vi "Close.vi"(8 "error in (no error)":errorcluster) -> (0 "error out":errorcluster)   [LabVIEW 2018, in "app_log.lvlib"]
doc: "Closes the reference to the log file.\n\nError handling\n- execute even if error at input\n- clear all errors (i.e. guaranteed that this VI will NOT generate an error of its own)\n- pass error in to error out"
uses:
  app_log.lvlib
  text_file/text_file.lvlib
panel:
  # "Development\ncontrols/indicators useful for development and testing, but which are not outputs of the VI"
  # "Input\nInputs to the VI"
  # "Output\nOutputs of the VI"
  # "Description\n\nBlank VI with error handling case. \n\nSummarize the use of this VI in this space."
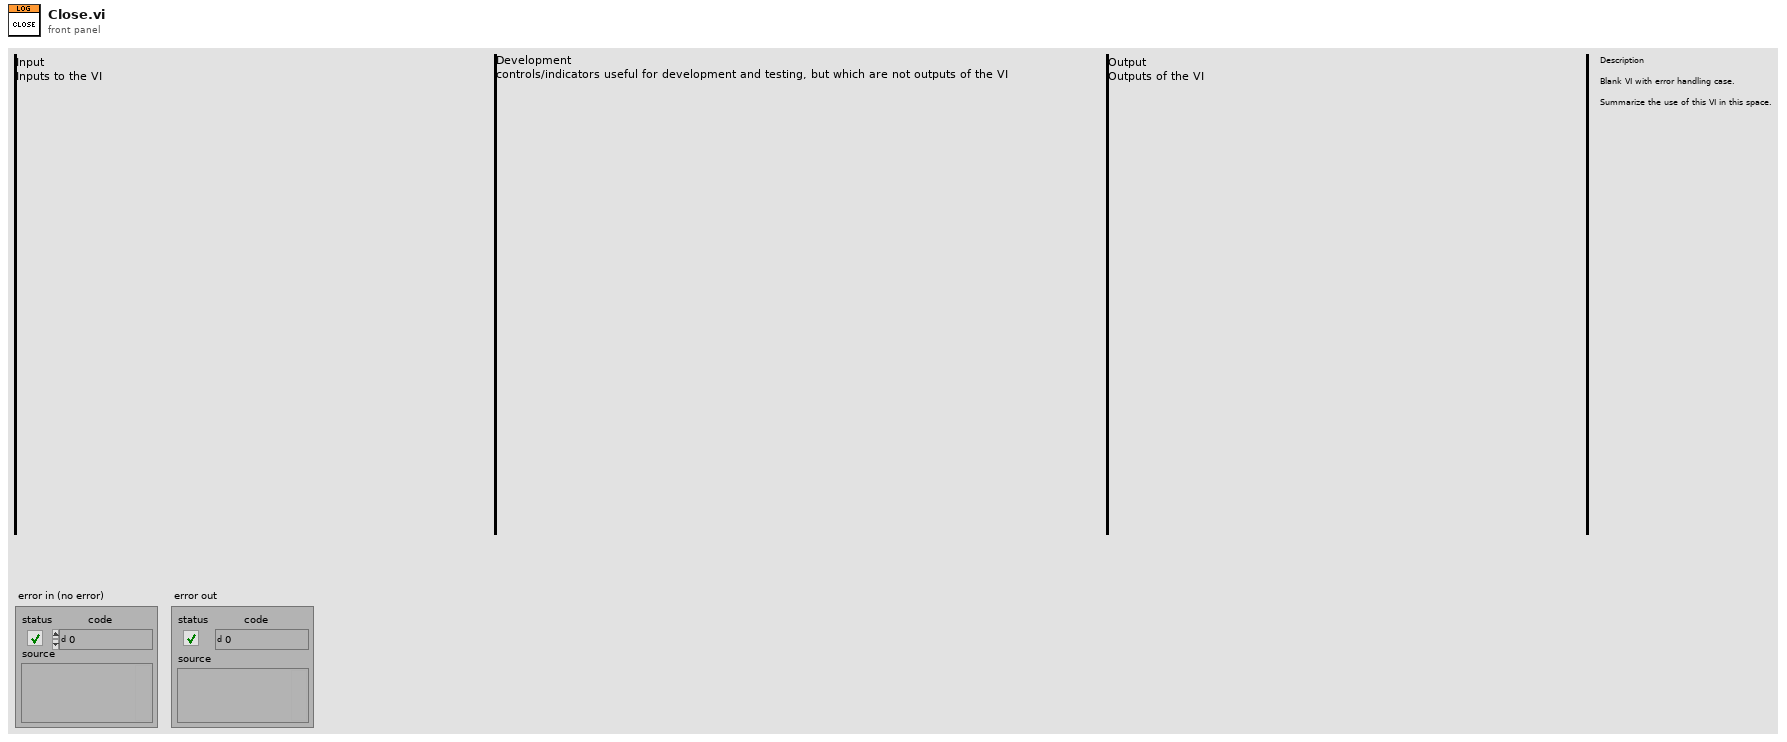
[diagram p1: front panel]
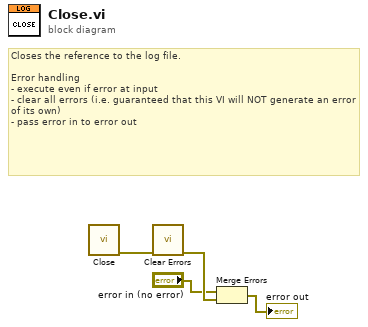
[diagram p0: block diagram]
diagram:
  # "Closes the reference to the log file.\n\nError handling\n- execute even if error at input\n- clear all errors (i.e. guaranteed that this VI will NOT generate an error of its own)\n- pass error in to error out"
  n1 = call "Close.vi"() -> ("error out"=w4:errorcluster)  [unwired: 11 in]
  n2 = call <vilib>:"Clear Errors.vi"("error in (no error)"=w4) -> ("error out"=w3:errorcluster)  [unwired: 5 in, 1 out]
  n3 = Merge Errors("error in (no error)", w3) -> (→"error out":errorcluster)
